vi "parseEMCY.vi"(8 "error in (no error)":errorcluster, 10 "emergency message":T1, 11 "MotorControllerClass in":refnum<class "MotorControllerClass.lvclass">) -> (0 "error out":errorcluster, 3 "MotorControllerClass out":refnum<class "MotorControllerClass.lvclass">)   [LabVIEW 2018, in "MotorControllerClass.lvclass"]
uses:
  MotorControllerClass.lvclass
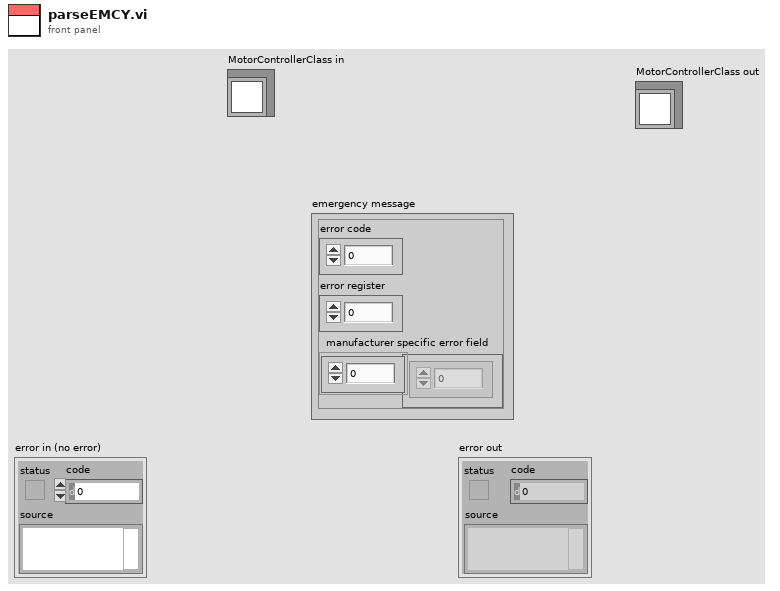
[diagram p1: front panel]
types:
  T1 = cluster{"error code":dbl, "error register":dbl, "manufacturer specific error field":dbl[]}
  T2 = typedef "TypeDef_MotorData.ctl" = cluster{" Velocity (RPM)":i32, " MotorTemp(C)":u8, " ControlTemp(C)":u8, " DcLinkVolt(V)":dbl, " ErrorCode":dbl, "IsAlive":bool, "motorStatus":cluster{"isReady":bool, "isOn":bool, "isOperEn":bool, "isFault":bool, "isVoltEn":bool, "targetReached":bool, "isWarning":bool}, "motorControllerState":u16}
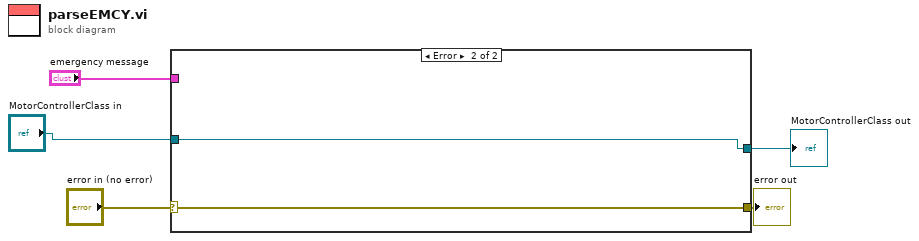
[diagram p0: block diagram]
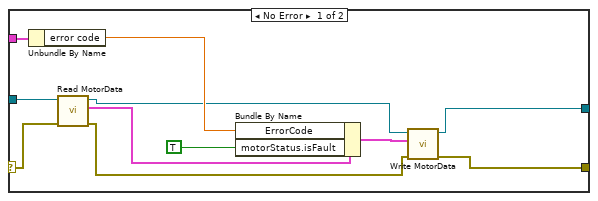
[diagram p2: hidden frame]
diagram:
  n1 = case shown="Error" "error in (no error)" {
    selector: "error in (no error)" -> [w10 w18]
    tunnel: [w7 w18] -> w4
    tunnel: "emergency message" -> [w16 _]
    tunnel: "MotorControllerClass in" -> [w12 w17]
    tunnel: [w6 w17] -> w1
    frame No Error {
      n2 = Unbundle By Name(w16) -> ("error code"=w15:dbl)
      n3 = call-dynamic "Read MotorData.vi"("error in (no error)"=w10, "MotorControllerClass in"=w12) -> ("error out"=w8:errorcluster, "MotorData"=w11:T2, "MotorControllerClass out"=w13:refnum<class "MotorControllerClass.lvclass">)  [unwired: 7 in]
      n4 = Bundle By Name(cluster=w11, "ErrorCode"=w15, "motorStatus.isFault"=TRUE) -> (w9:T2)
      n5 = call-dynamic "Write MotorData.vi"("error in (no error)"=w8, "MotorData"=w9, "MotorControllerClass in"=w13) -> ("error out"=w7:errorcluster, "MotorControllerClass out"=w6:refnum<class "MotorControllerClass.lvclass">)  [unwired: 7 in]
    }
    frame Error {
    }
  }
  "error out" <- w4
  "MotorControllerClass out" <- w1
